vi "setConnectionReport.vi"(9 "string":string, 11 "Type of Message":u16(ring) items=["connectedMsg", "disconnectedMsg", "openVIRefMsg", "closeVIRefMsg"]) -> ()   [LabVIEW 2010]
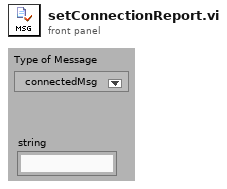
[diagram p1: front panel]
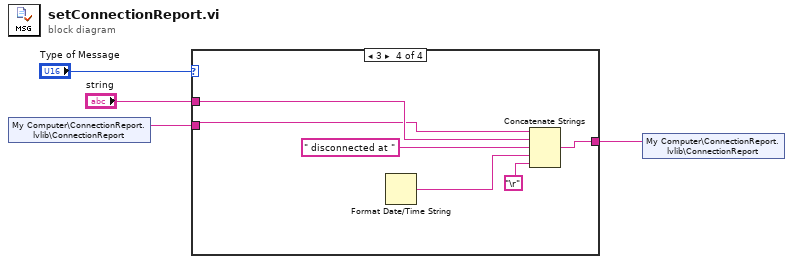
[diagram p0: block diagram]
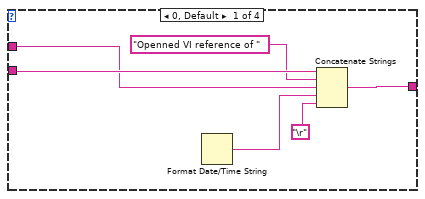
[diagram p2: hidden frame]
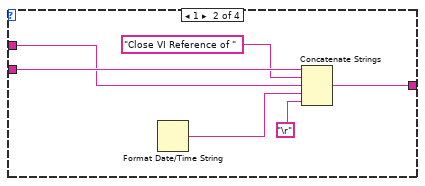
[diagram p3: hidden frame]
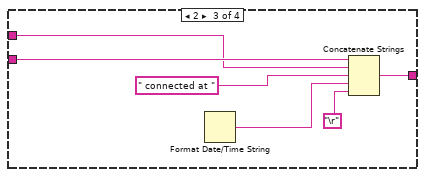
[diagram p4: hidden frame]
diagram:
  n1 = shared-variable "My Computer\\ConnectionReport.lvlib\\ConnectionReport"() -> (w3:string)  [unwired: 1 in, 1 out]
  n2 = case shown="3" "Type of Message" {
    tunnel: w3 -> [w8 w14 w19 w24]
    tunnel: [w7 w13 w17 w23] -> w2
    tunnel: "string" -> [w6 w12 w18 w25]
    frame 0, Default {
      n3 = Format Date/Time String() -> (date/time string=w10:string)  [unwired: 3 out]
      n4 = Concatenate Strings(w8, "Openned VI reference of " ("string"), w6, w10, "\r") -> (w7:string)
    }
    frame 1 {
      n5 = Format Date/Time String() -> (date/time string=w15:string)  [unwired: 3 out]
      n6 = Concatenate Strings(w14, "Close VI Reference of " ("string"), w12, w15, "\r") -> (w13:string)
    }
    frame 2 {
      n7 = Format Date/Time String() -> (date/time string=w21:string)  [unwired: 3 out]
      n8 = Concatenate Strings(w19, w18, " connected at " ("string"), w21, "\r") -> (w17:string)
    }
    frame 3 {
      n9 = Format Date/Time String() -> (date/time string=w27:string)  [unwired: 3 out]
      n10 = Concatenate Strings(w24, w25, " disconnected at " ("string"), w27, "\r") -> (w23:string)
    }
  }
  n11 = shared-variable "My Computer\\ConnectionReport.lvlib\\ConnectionReport"(w2) -> ()  [unwired: 1 in, 1 out]
